vi "Send Startup Notification.vi"(8 "error in (no error)":errorcluster, 11 "VolatusCore in":refnum<class "VolatusCore.lvclass">) -> (0 "error out":errorcluster, 3 "VolatusCore out":refnum<class "VolatusCore.lvclass">)   [LabVIEW 2020, in "Volatus.lvlib" / "VolatusCore.lvclass"]
uses:
  VolatusCore.lvclass
  Startup Notification.ctl
  App/App.lvclass
  Core APIs.ctl
  VolatusAPI/VolatusAPI.lvclass
  Event API/EventAPI.lvclass
  ConfigAPI/ConfigAPI.lvclass
  VolatusCore.lvclass/VolatusCore.ctl
  Volatus.lvlib
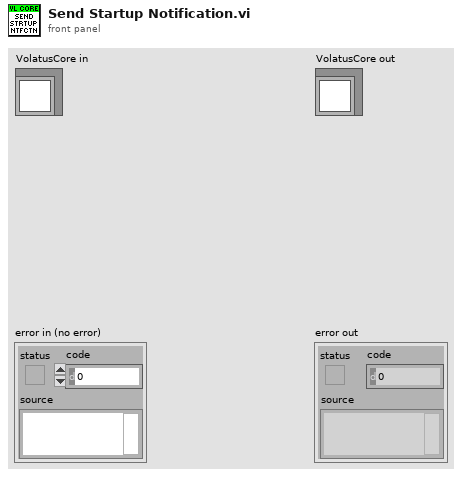
[diagram p1: front panel]
types:
  T1 = typedef "Volatus.lvlib/VolatusCore.lvclass/Startup Notification.ctl" = cluster{"Start":bool, "App":refnum<class "App.lvclass">, "Core APIs":T2}
  T2 = typedef "Volatus.lvlib/Core APIs.ctl" = cluster{"Volatus":refnum<class "VolatusAPI.lvclass">, "Event":refnum<class "EventAPI.lvclass">, "Config":refnum<class "ConfigAPI.lvclass">}
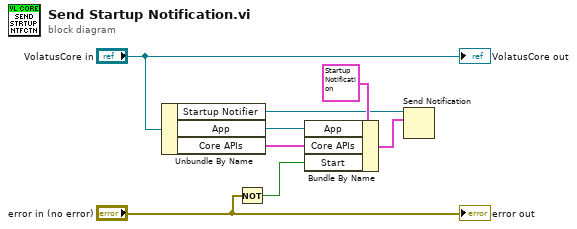
[diagram p0: block diagram]
diagram:
  n1 = Unbundle By Name("VolatusCore in") -> ("Startup Notifier"=w4:refnum<notifier>, "App"=w5:refnum<class "App.lvclass">, "Core APIs"=w1:T2)
  n2 = Not(x="error in (no error)") -> (.not. x?=w2:bool)
  n3 = Bundle By Name(cluster=T1 {"Start"=FALSE, "App"=refnum, "Core APIs"={"Volatus"=refnum, "Event"=refnum, "Config"=refnum}} ("Startup Notification"), "App"=w5, "Core APIs"=w1, "Start"=w2) -> (w3:T1)
  n4 = Send Notification(notification=w3, notifier=w4) -> ()  [unwired: 1 in, 2 out]
  "error out" <- "error in (no error)"
  "VolatusCore out" <- "VolatusCore in"
